vi "AcommandQueues.vi"(8 "ErrorIn":errorcluster, 9 "ACommandIn":T1, 10 "ACommandQueuesAction":T2=enum."Get", 11 "AThreads":T3[](array[typedef])) -> (0 "ErrorOut":errorcluster, 1 "ACommandOut":T1)   [LabVIEW 2019]
uses:
  AThreads.ctl
  ACommandQueuesAction.ctl
  ACommand.ctl
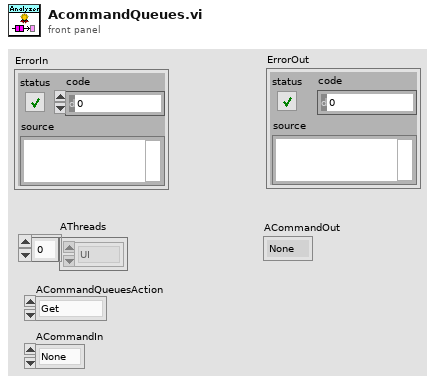
[diagram p1: front panel]
types:
  T1 = typedef "ACommand.ctl" = enum16{"None", "Start", "Stop", "Restart", "SendFilesData", "DeleteAllData"}
  T2 = typedef "ACommandQueuesAction.ctl" = enum16{"Initialize", "Set", "Get", "ReleaseAll"}
  T3 = typedef "AThreads.ctl" = enum16{"UI", "analyzeAccelerationData", "aquireAccelerationData", "communicateWebServices", "TDMSmanager", "aquireTachoSignal"}
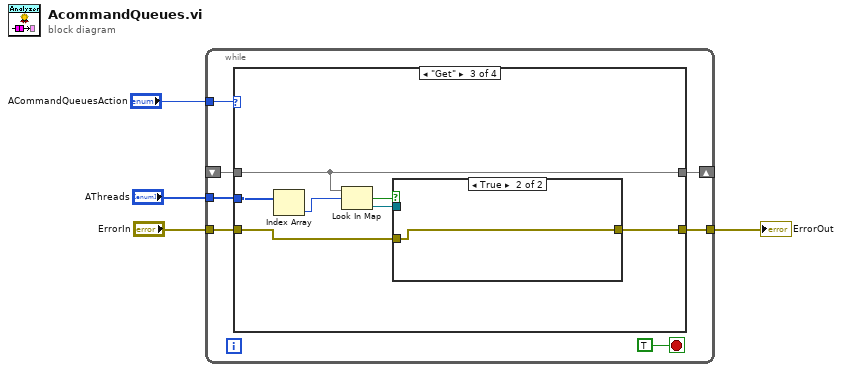
[diagram p0: block diagram]
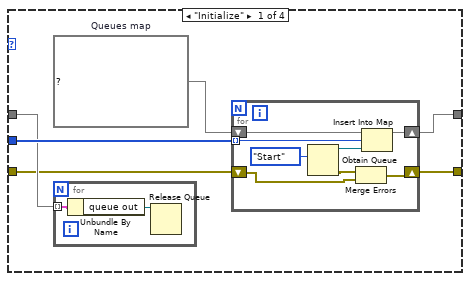
[diagram p2: hidden frame]
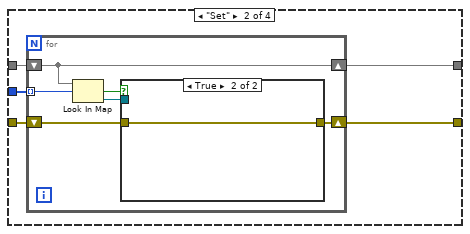
[diagram p3: hidden frame]
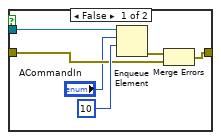
[diagram p4: hidden frame]
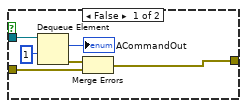
[diagram p5: hidden frame]
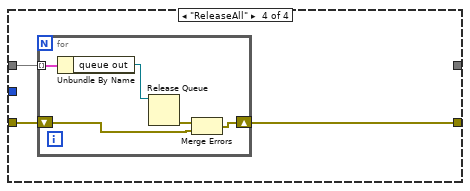
[diagram p6: hidden frame]
diagram:
  n1 = while {
    tunnel: "ACommandQueuesAction" -> [w11]
    tunnel: "AThreads" -> [w10]
    shift-right: [w8] -> _
    shift-left: _ -> [w6]
    tunnel: "ErrorIn" -> [w9]
    tunnel: [w5] -> w4
    stop <- TRUE stop-if-true
    n2 = case shown="\"Get\"" w11 {
      tunnel: w10 -> [w17 w31 w50 _]
      tunnel: w9 -> [w12 w28 w47 w61]
      tunnel: [w16 w29 w52 _] -> w8
      tunnel: w6 -> [w13 w32 w52 w62]
      tunnel: [w14 w30 w48 w60] -> w5
      frame "Initialize" {
        w15 = map{T3, refnum<queue>} {}  # Queues map
        n3 = for {
          tunnel: w13 -> [w19] mode=indexing
          n4 = Unbundle By Name(w19) -> ("queue out"=w18:refnum<queue>)
          n5 = Release Queue(queue=w18) -> ()  [unwired: 2 in, 3 out]
        }
        n6 = for {
          tunnel: w17 -> [w26] mode=indexing
          shift-right: [w23] -> w14
          shift-left: w12 -> [w22]
          shift-right: [w25] -> w16
          shift-left: w15 -> [w27]
          n7 = Obtain Queue(element data type=ACommand."Start" ("AnalyzerCommand")) -> (queue out=w20:refnum<queue>, error out=w24:errorcluster)  [unwired: 4 in, 1 out]
          n8 = Merge Errors(w24, w22) -> (w23:errorcluster)
          n9 = Insert Into Map(map in=w27, key=w26, value=w20) -> (map out=w25:map{T3, refnum<queue>})  [unwired: 2 out]
        }
      }
      frame "Set" {
        n10 = for {
          tunnel: w31 -> [w38] mode=indexing
          shift-right: [w34] -> w30
          shift-left: w28 -> [w35]
          shift-right: [w36] -> w29
          shift-left: w32 -> [w36]
          n11 = Look In Map(map=w36, key=w38) -> (key not found?=w33:bool, value=w37:refnum<queue>)  [unwired: 1 in]
          n12 = case shown="True" w33 {
            tunnel: w37 -> [w44 _]
            tunnel: w35 -> [w41 w45]
            tunnel: [w39 w45] -> w34
            frame False {
              n13 = Enqueue Element(queue=w44, element="ACommandIn", timeout in ms (-1)=10) -> (error out=w42:errorcluster)  [unwired: 1 in, 2 out]
              n14 = Merge Errors(w42, w41) -> (w39:errorcluster)
            }
            frame True {
            }
          }
        }
      }
      frame "Get" {
        n15 = Index Array(array=w50) -> (element=w49:T3)  [unwired: 1 in]
        n16 = Look In Map(map=w52, key=w49) -> (key not found?=w46:bool, value=w51:refnum<queue>)  [unwired: 1 in]
        n17 = case shown="True" w46 {
          tunnel: w51 -> [w57 _]
          tunnel: [w55 w59] -> w48
          tunnel: w47 -> [w54 w59]
          frame False {
            n18 = Dequeue Element(queue=w57, timeout in ms (-1)=1) -> (element=→"ACommandOut":T1, error out=w58:errorcluster)  [unwired: 1 in, 2 out]
            n19 = Merge Errors(w58, w54) -> (w55:errorcluster)
          }
          frame True {
          }
        }
      }
      frame "ReleaseAll" {
        n20 = for {
          tunnel: w62 -> [w67] mode=indexing
          shift-right: [w64] -> w60
          shift-left: w61 -> [w63]
          n21 = Unbundle By Name(w67) -> ("queue out"=w66:refnum<queue>)
          n22 = Release Queue(queue=w66) -> (error out=w65:errorcluster)  [unwired: 2 in, 2 out]
          n23 = Merge Errors(w65, w63) -> (w64:errorcluster)
        }
      }
    }
  }
  "ErrorOut" <- w4
